vi "Query Ring String from Value.vi"(8 "error in (no error)":errorcluster, 10 "AI.MeasType":i32, 11 "Ring Ref":refnum<vi>) -> (0 "error out":errorcluster, 3 "String":string)   [LabVIEW 2021, in "XNET-CAN-Signal-Logger.lvlib"]
uses:
  XNET-CAN-Signal-Logger.lvlib
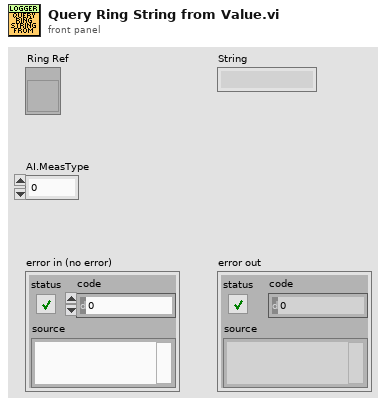
[diagram p1: front panel]
types:
  T1 = typedef "LVStringsAndValuesArrayTypeDef_I32.ctl" = cluster{"String":string, "Value":i32}[]
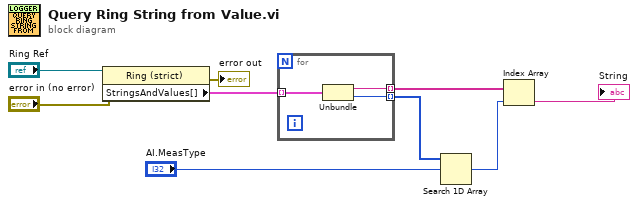
[diagram p0: block diagram]
diagram:
  n1 = property on="Property Node" class="Ring (strict)"(reference="Ring Ref", error in="error in (no error)") -> (error out=→"error out":errorcluster, "StringsAndValues[]"=w4:T1)  [unwired: 1 out]
  n2 = for {
    tunnel: w4 -> [w12] mode=indexing
    tunnel: [w11] -> w7 mode=indexing
    tunnel: [w10] -> w5 mode=indexing
    n3 = Unbundle(w12) -> ("String"=w11:string, "Value"=w10:i32)
  }
  n4 = Search 1D Array(1D array=w5, element="AI.MeasType") -> (index of element=w8:i32)  [unwired: 1 in]
  n5 = Index Array(array=w7, index=w8) -> (element=→"String":string)
